vi "TFTP Get File.vi"(5 "net address":string, 6 "Binary (T)":bool=TRUE, 7 "timeout ms (1000)":i32=1000, 8 "error in (no error)":errorcluster, 9 "local path":path, 10 "remote path":string, 11 "Host":string) -> (0 "error out":errorcluster, 2 "Status":bool, 3 "File Length":i32)   [LabVIEW 2013]
doc: "Connects to an TFTP server and copies a single file to the local machine."
panel:
  out "local port":u16
  out "file error":errorcluster
  out "server port":u16
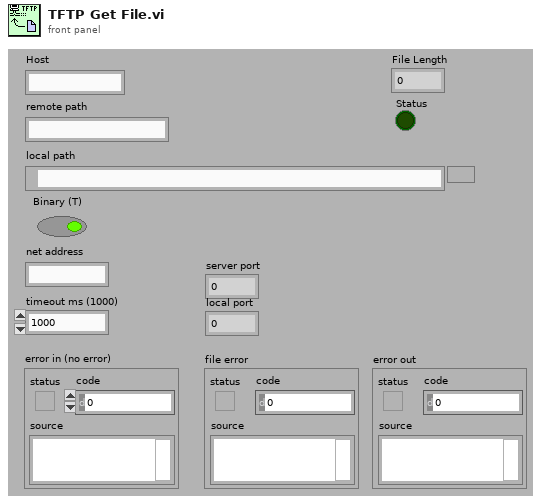
[diagram p1: front panel]
types:
  T1 = enum16{"open", "replace", "create", "open or create", "replace or create", "replace or create with confirmation"}
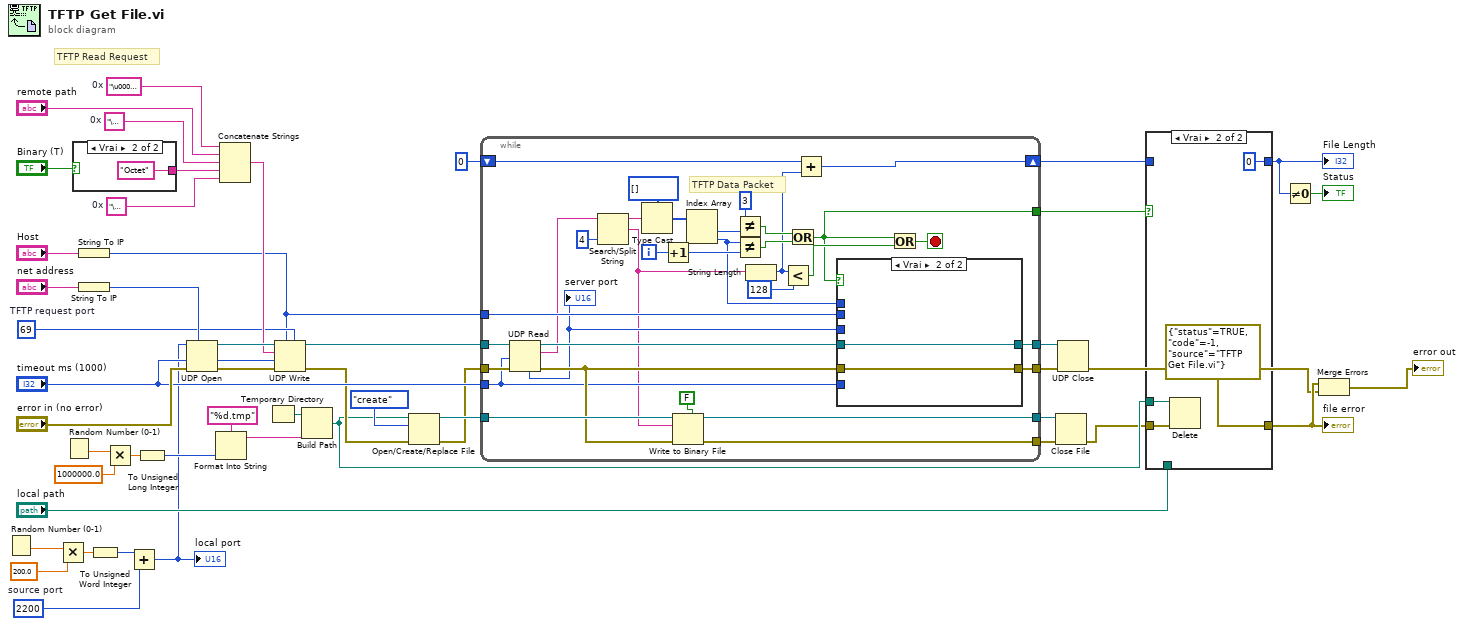
[diagram p0: block diagram]
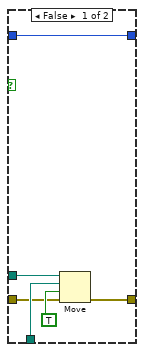
[diagram p2: hidden frame]
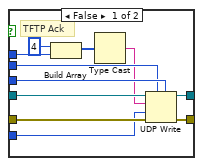
[diagram p3: hidden frame]
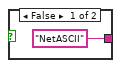
[diagram p4: hidden frame]
diagram:
  w7 = u16 2200  # source port
  w41 = "\u0000"  # 0x
  w43 = "\u0000"  # 0x
  w45 = "\u0000\u0001"  # 0x
  w36 = u16 69  # TFTP request port
  # "TFTP Read Request"
  n1 = Random Number (0-1)() -> (number: 0 to 1=w9:dbl)
  n2 = Multiply(x=w9, y=200.0) -> (x*y=w11:dbl)
  n3 = Random Number (0-1)() -> (number: 0 to 1=w27:dbl)
  n4 = case shown="Vrai" "Binary (T)" {
    tunnel: ["NetASCII" "Octet"] -> w42
    frame False {
    }
    frame True {
    }
  }
  n5 = String To IP(1:"Host") -> (0:w35:u32)
  n6 = String To IP(1:"net address") -> (0:w37:u32)
  n7 = To Unsigned Word Integer(number=w11) -> (unsigned 16bit integer=w8:u16)
  n8 = Multiply(x=w27, y=1000000.0) -> (x*y=w25:dbl)
  n9 = Add(x=w8, y=w7) -> (x+y=w6:u16)
  "local port" <- w6
  n10 = To Unsigned Long Integer(number=w25) -> (unsigned 32bit integer=w23:u32)
  n11 = UDP Open(7:w37, 8:"error in (no error)", 9:"timeout ms (1000)", 11:w6) -> (port=w48:refnum<k16>, 0:w47:errorcluster)  [unwired: 2 out]
  n12 = Format Into String(format string="%d.tmp", w23) -> (resulting string=w20:string)  [unwired: 2 in, 1 out]
  n13 = Concatenate Strings(w45, "remote path", w43, w42, w41) -> (w40:string)
  n14 = Temporary Directory() -> (w21:path)
  n15 = UDP Write(address=w35, port or service name=w36, connection ID=w48, data in=w40, 8:w47, 9:"timeout ms (1000)") -> (error out=w24:errorcluster, 3:w32:refnum<k16>)
  n16 = Build Path(base path=w21, name or relative path=w20) -> (appended path=w15:path)
  n17 = Open/Create/Replace File(file path (use dialog)=w15, error in=w24, operation (0:open)=T1."create") -> (refnum out=w31:refnum<file>, error out=w30:errorcluster)  [unwired: 4 out]
  n18 = while {
    tunnel: w32 -> [w84]
    tunnel: w30 -> [w83]
    tunnel: w31 -> [w72]
    tunnel: w35 -> [w66]
    tunnel: "timeout ms (1000)" -> [w64]
    tunnel: [w63] -> w29
    tunnel: [w62] -> w28
    tunnel: [w61] -> w18
    tunnel: [w60] -> w33
    tunnel: [w59] -> w17
    shift-right: [w52] -> w12
    shift-left: 0 -> [w53]
    i -> [w76]
    stop <- w69 stop-if-true
    # "TFTP Data Packet"
    n19 = UDP Read(connection ID=w84, timeout ms (25000)=w64, 8:w83) -> (data out=w58:string, error out=w67:errorcluster, 3:w68:refnum<k16>, 4:w57:u16)  [unwired: 2 out]
    "server port" <- w57
    n20 = Search/Split String(string=w58, offset (0)=4) -> (substring before match=w80:string, match + rest of string=w56:string)  [unwired: 2 out]
    n21 = Type Cast(type=u16[] [], x=w80) -> (*(type *) &x=w79:u16[])
    n22 = Increment(x=w76) -> (x+1=w75:i32)
    n23 = Write to Binary File(file (use dialog)=w72, data=w56, error in=w67, 5:FALSE ("prepend array or string size? (T)")) -> (refnum out=w63:refnum<file>, error out=w62:errorcluster)  [unwired: 3 out]
    n24 = Index Array(array=w79) -> (element #1=w78:u16, element #2=w65:u16)  [unwired: 2 in]
    n25 = Not Equal?(x=u16 3, y=w78) -> (x != y?=w73:bool)
    n26 = Not Equal?(x=w65, y=w75) -> (x != y?=w74:bool)
    n27 = String Length(string=w56) -> (length=w54:i32)
    n28 = Less?(x=w54, y=128) -> (x < y?=w70:bool)
    n29 = Or(x=w73, y=w74) -> (x .or. y?=w59:bool)
    n30 = Add(x=w53, y=w54) -> (x+y=w52:i32)
    n31 = case shown="Vrai" w59 {
      tunnel: w68 -> [w95 w97]
      tunnel: w67 -> [w94 w96]
      tunnel: w57 -> [w93 _]
      tunnel: w66 -> [w92 _]
      tunnel: w65 -> [w90 _]
      tunnel: w64 -> [w88 _]
      tunnel: [w87 w96] -> w61
      tunnel: [w86 w97] -> w60
      frame False {
        # "TFTP Ack"
        n32 = Build Array(u16 4, w90) -> (w89:u16[])
        n33 = Type Cast(x=w89) -> (*(type *) &x=w85:string)  [unwired: 1 out]
        n34 = UDP Write(address=w92, port or service name=w93, connection ID=w95, data in=w85, 8:w94, 9:w88) -> (error out=w87:errorcluster, 3:w86:refnum<k16>)
      }
      frame True {
      }
    }
    n35 = Or(x=w59, y=w70) -> (x .or. y?=w69:bool)
  }
  n36 = Close File(refnum=w29, error in=w28) -> (error out=w14:errorcluster)  [unwired: 1 out]
  n37 = UDP Close(connection ID=w33, 8:w18) -> (error out=w2:errorcluster)  [unwired: 1 out]
  n38 = case shown="Vrai" w17 {
    tunnel: "local path" -> [w101 _]
    tunnel: w15 -> [w103 w107]
    tunnel: w14 -> [w100 w106]
    tunnel: [w99 errorcluster {"status"=TRUE, "code"=-1, "source"="TFTP Get File.vi"} ("error out")] -> w3
    tunnel: w12 -> [w98 _]
    tunnel: [w98 0] -> w5
    frame False {
      n39 = Move(source path=w103, error in=w100, 9:TRUE ("overwrite (F)"), 10:w101) -> (error out=w99:errorcluster)  [unwired: 3 out]
    }
    frame True {
      n40 = Delete(path (use dialog)=w107, error in=w106) -> ()  [unwired: 6 out]
    }
  }
  "file error" <- w3
  "File Length" <- w5
  n41 = Not Equal To 0?(x=w5) -> (x != 0?=→"Status":bool)
  n42 = Merge Errors(w3, w2) -> (→"error out":errorcluster)
